vi "To Serial Form.vi"(6 "Serial Version":T1, 10 "Serializer in":refnum<class "Serializer.lvclass">, 11 "U16 in":refnum<class "U16.lvclass">) -> (0 "error out":errorcluster, 2 "Serializer out":refnum<class "Serializer.lvclass">, 3 "U16 out":refnum<class "U16.lvclass">)   [LabVIEW 2014, in "Base Data Class.lvlib" / "U16.lvclass"]
uses:
  U16.lvclass
  <vilib>/NI/AQ Character Lineator/Serializer/Serializer.lvclass
  <vilib>/NI/AQ Character Lineator/Serialization Common/Serial Version.ctl
  U16.lvclass/U16.ctl
  <vilib>/NI/AQ Character Lineator/Serializable/Insert UInt16.vi
  <vilib>/NI/AQ Character Lineator/Serializer/Insert UInt16.vi
  <vilib>/NI/AQ Character Lineator/Serializer/Read Include Default Values.vi
  Data.lvclass
  <vilib>/NI/AQ Character Lineator/Serializable/Serializable.lvclass
  <vilib>/NI/AQ Character Lineator/Serialization Common/Serialization Common.lvlib
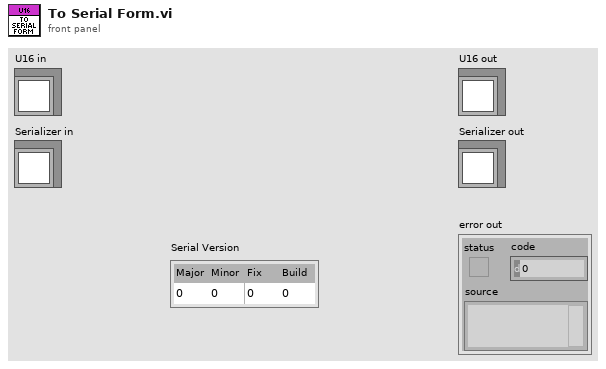
[diagram p1: front panel]
types:
  T1 = typedef "Serialization Common.lvlib/Serial Version.ctl" = cluster{"Major":u16, "Minor":u16, "Fix":u16, "Build":u16}
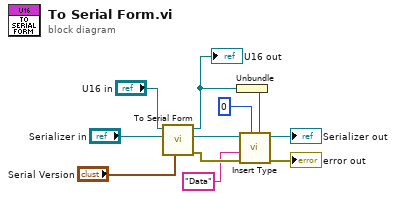
[diagram p0: block diagram]
diagram:
  n1 = call-parent "To Serial Form.vi"("Serial Version"="Serial Version", "Serializer in"="Serializer in", "Data in"="U16 in") -> ("error out"=w3:errorcluster, "Serializer out"=w7:refnum<class "Serializer.lvclass">, "Data out"=w6:refnum<class "U16.lvclass">)  [unwired: 6 in]
  "U16 out" <- w6
  n2 = Unbundle(w6) -> (w5:u16)
  n3 = call-poly <vilib>:"Insert Type.vi"("Integer"=w5, "Default Value"=u16 0, "error in (no error)"=w3, "Name"="Data", "Serializer in"=w7) -> ("error out"=→"error out":errorcluster, "Serializer out"=→"Serializer out":refnum<class "Serializer.lvclass">)  [unwired: 5 in]
